vi "X_plant.vi"(4 "u":dbl format="%#_13g") -> (1 "y":dbl)   [LabVIEW 2019]
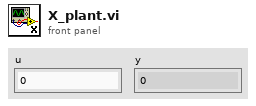
[diagram p1: front panel]
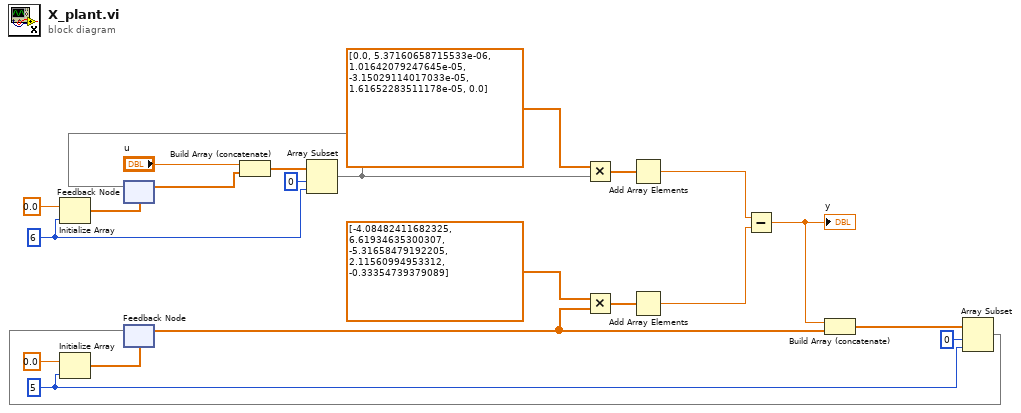
[diagram p0: block diagram]
diagram:
  w6 = 5 ("dimension size")
  w17 = 6 ("dimension size")
  n1 = Initialize Array(0.0 ("element"), w17) -> (w16:dbl[])
  n2 = Initialize Array(0.0 ("element"), w6) -> (w9:dbl[])
  n3 = feedback #1(w16) -> (w21:dbl[])
  n4 = feedback #2(w9) -> (w12:dbl[])
  n5 = Build Array (concatenate)("u", w21) -> (w20:dbl[])
  n6 = Array Subset(array=w20, index=0, length=w17) -> (w15:dbl[])
  n7 = feedback-in #1(w15) -> ()
  n8 = Multiply(x=dbl[] [0.0, 5.37160658715533e-06, 1.01642079247645e-05, -3.15029114017033e-05, 1.61652283511178e-05, 0.0] ("Qd"), y=w15) -> (x*y=w4:dbl[])
  n9 = Multiply(x=dbl[] [-4.08482411682325, 6.61934635300307, -5.31658479192205, 2.11560994953312, -0.33354739379089] ("Qd"), y=w12) -> (x*y=w11:dbl[])
  n10 = Add Array Elements(numeric array=w4) -> (sum=w3:dbl)
  n11 = Add Array Elements(numeric array=w11) -> (sum=w2:dbl)
  n12 = Subtract(x=w3, y=w2) -> (x-y=w1:dbl)
  "y" <- w1
  n13 = Build Array (concatenate)(w1, w12) -> (w8:dbl[])
  n14 = Array Subset(array=w8, index=0, length=w6) -> (w5:dbl[])
  n15 = feedback-in #2(w5) -> ()
